vi "Filter.vi"(11 "Input":sgl) -> (3 "Output":sgl)   [LabVIEW 2016, in "DCM-Classes.lvlib" / "DCM - RT.lvclass"]
uses:
  DCM - RT.lvclass
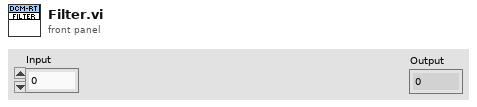
[diagram p1: front panel]
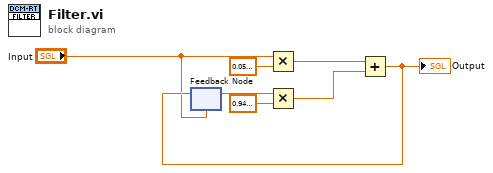
[diagram p0: block diagram]
diagram:
  n1 = feedback #1("Input") -> (w7:sgl)
  n2 = Multiply(x="Input", y=sgl 0.05) -> (x*y=w4:sgl)
  n3 = Multiply(x=w7, y=sgl 0.95) -> (x*y=w3:sgl)
  n4 = Add(x=w4, y=w3) -> (x+y=w2:sgl)
  "Output" <- w2
  n5 = feedback-in #1(w2) -> ()
